vi "Display hologram.vi"(0 "CGH in":u8[][](array[numeric])=array512x512[262144 elements], 1 "CUDA/SLM error in":errorcluster) -> (2 "return":i32, 3 "CGH out":u8[][](array[numeric]), 4 "CUDA/SLM error out":errorcluster)   [LabVIEW 2012]
uses:
  C/x64/Release_PCIeSLM/GenerateHologramCUDA.dll
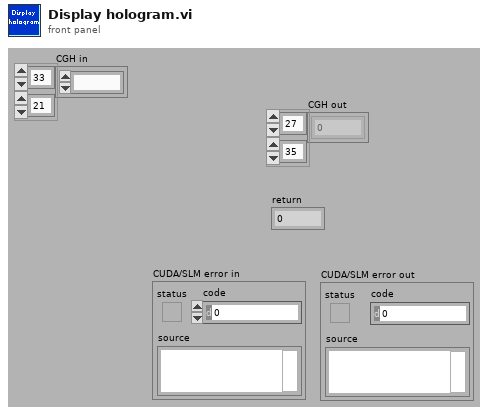
[diagram p1: front panel]
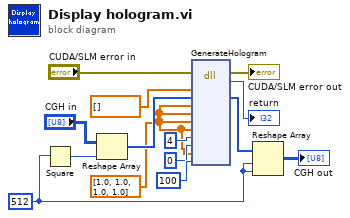
[diagram p0: block diagram]
diagram:
  w1 = sgl[] [1.0, 1.0, 1.0, 1.0] ("x")
  w8 = 512 ("SLM size")
  n1 = Square(x=w8) -> (x^2=w9:i32)
  n2 = Reshape Array("CGH in", w9) -> (w7:u8[])
  n3 = dll-call lib="D:/Dropbox/CUDA/GenerateHologramCUDA/C/x64/Release_PCIeSLM/GenerateHologramCUDA.dll" fn="GenerateHologram"(error in="CUDA/SLM error in", "V"=sgl[] [], "h_pSLM"=w7, "x"=w1, "y"=w1, "z"=w1, "spot_amplitudes"=w1, "N_spots"=4, "N_iterations"=0, "weights"=w1, "method"=100) -> (error out=→"CUDA/SLM error out":errorcluster, "return"=→"return":i32, "h_pSLM"=w4:u8[])  [unwired: 5 in, 7 out]
  n4 = Reshape Array(w4, w8, w8) -> (→"CGH out":u8[][])
